vi "Y_H_change_value.vi"(8 "error in (no error)":errorcluster, 11 "Y_H_in":refnum<class "Y_H.lvclass">) -> (0 "error out":errorcluster, 3 "Y_H_out":refnum<class "Y_H.lvclass">)   [LabVIEW 2019, in "Y_H.lvclass"]
uses:
  Y_H.lvclass
  Y_H.lvclass/Y_H.ctl
  ctl/Y_H_state.ctl
  Timer Delay/Timers.lvlib
panel:
  in  "setpoint":T1(slide) caption="oC" scale=0.0..500.0 scale format="%#_5g"
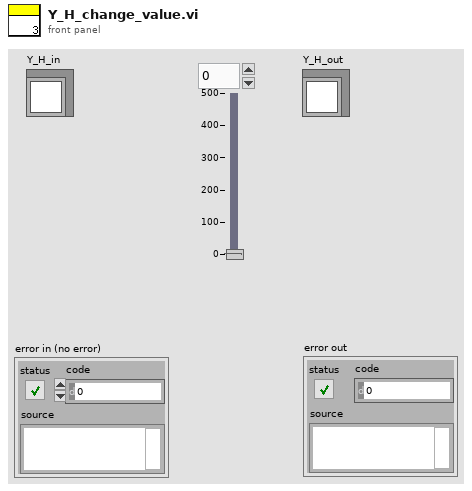
[diagram p1: front panel]
types:
  T1 = cluster{"Numeric":dbl, "Numeric":dbl, "Numeric":dbl}
  T2 = typedef "control.lvlib/Y_source.ctl" = enum8{"initialize", "local disabled", "local hand", "hand", "auto", "dist"}
  T3 = typedef "Y_H.lvclass/Y_H_state.ctl" = enum16{"init", "value change", "value not changed"}
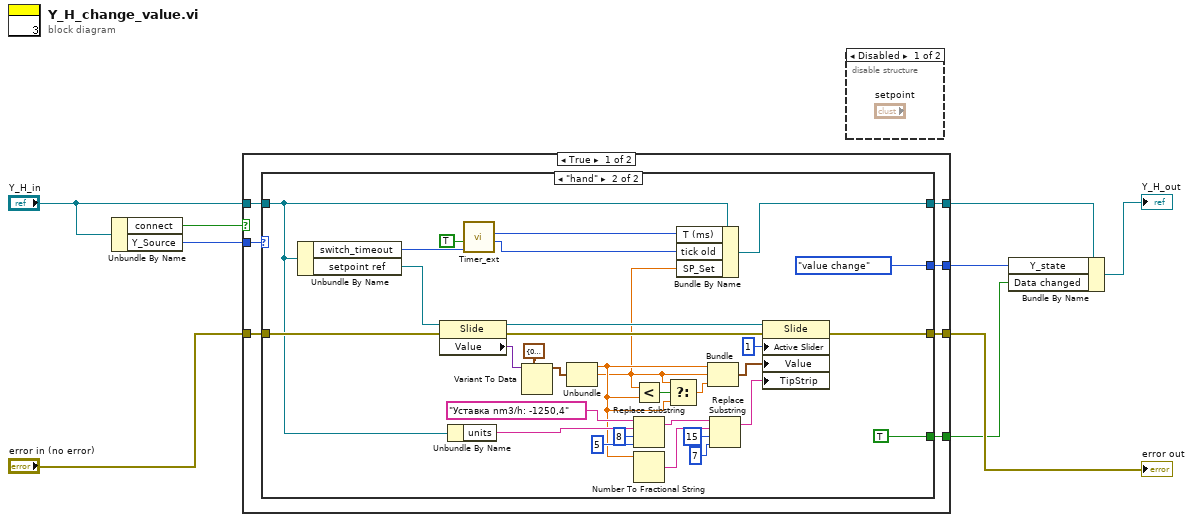
[diagram p0: block diagram]
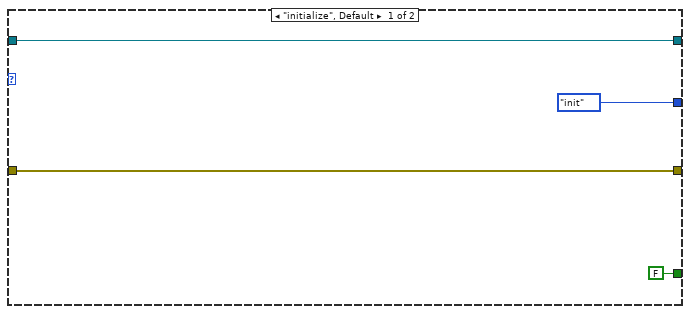
[diagram p2: hidden frame]
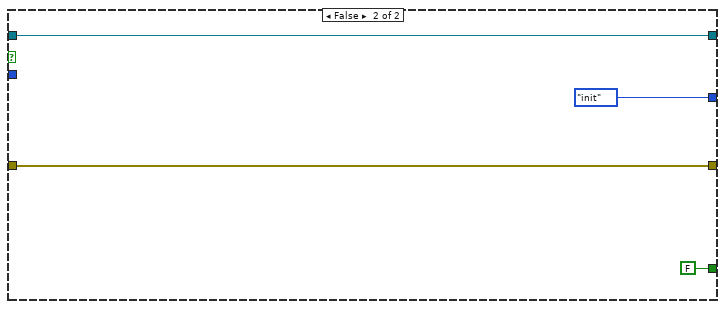
[diagram p3: hidden frame]
diagram:
  n1 = Unbundle By Name("Y_H_in") -> ("connect"=w6:bool, "Y_Source"=w5:T2)
  n2 = case shown="True" w6 {
    tunnel: w5 -> [w16 _]
    tunnel: [w15 Y_H_state."init" ("switch_state")] -> w1
    tunnel: "error in (no error)" -> [w13 w54]
    tunnel: "Y_H_in" -> [w14 w52]
    tunnel: [w12 w54] -> w7
    tunnel: [w11 FALSE] -> w4
    tunnel: [w10 w52] -> w2
    frame True {
      n3 = case shown="\"hand\"" w16 {
        tunnel: [Y_H_state."init" ("switch_state") Y_H_state."value change" ("switch_state")] -> w15
        tunnel: w14 -> [w17 w22]
        tunnel: w13 -> [w19 w51]
        tunnel: [w19 w49] -> w12
        tunnel: [FALSE TRUE] -> w11
        tunnel: [w17 w23] -> w10
        frame "initialize", Default {
          # "local hand"
        }
        frame "hand" {
          # "local hand"
          n4 = Unbundle By Name(w22) -> ("switch_timeout"=w27:u32, "setpoint ref"=w38:refnum<vi>)
          n5 = property on="Property Node" class="Slide"(reference=w38, error in=w51) -> (reference out=w37:refnum<vi>, error out=w36:errorcluster, "Value"=w31:variant)
          n6 = Unbundle By Name(w22) -> ("units"=w35:string)
          n7 = call "Timer_ext.vi"("ms"=w27, "Load"=TRUE) -> ("tick"=w24:u32, "t ms"=w25:u32)  [unwired: 7 in, 1 out]
          n8 = Variant To Data(type=cluster{"SP":dbl, "SP_Set":dbl, "SP":dbl} {"SP"=0.0, "SP_Set"=0.0, "SP"=0.0} ("output cluster"), Variant=w31) -> (data=w30:cluster{"SP":dbl, "SP_Set":dbl, "SP":dbl})  [unwired: 1 in, 1 out]
          n9 = Unbundle(w30) -> ("SP"=w29:dbl, "SP_Set"=w21:dbl)  [unwired: 1 out]
          n10 = Less?(x=w21, y=w29) -> (x < y?=w34:bool)
          n11 = Replace Substring(2:5 ("length (len. of substring)"), 3:8 ("offset (0)"), 4:w35, 5:"Уставка nm3/h: -1250,4") -> (1:w41:string)  [unwired: 1 out]
          n12 = Number To Fractional String(number=w29) -> (F-format string=w40:string)  [unwired: 3 in]
          n13 = Select(t=w21, s=w34, f=w29) -> (s? t:f=w33:dbl)
          n14 = Bundle By Name(cluster=w22, "T (ms)"=w25, "tick old"=w24, "SP_Set"=w21) -> (w23:refnum<class "Y_H.lvclass">)
          n15 = Bundle("SP"=w29, "SP_Set"=w21, "SP"=w33) -> (w28:cluster{"SP":dbl, "SP_Set":dbl, "SP":dbl})  [unwired: 1 in]
          n16 = Replace Substring(2:7 ("length (len. of substring)"), 3:15 ("offset (0)"), 4:w40, 5:w41) -> (1:w39:string)  [unwired: 1 out]
          n17 = property on="Property Node" class="Slide"(reference=w37, error in=w36, "Active Slider"=1, "Value"=w28, "TipStrip"=w39) -> (error out=w49:errorcluster)  [unwired: 1 out]
        }
      }
    }
    frame False {
    }
  }
  "error out" <- w7
  n18 = disable-structure shown="Disabled" {
    frame Disabled {
    }
    frame Enabled {
    }
  }
  n19 = Bundle By Name(cluster=w2, "Y_state"=w1, "Data changed"=w4) -> (→"Y_H_out":refnum<class "Y_H.lvclass">)
